vi "Add to Query.vi"(8 "error in (no error)":errorcluster, 9 "value":string, 10 "key":string, 11 "URI in":refnum<class "URI.lvclass">) -> (0 "error out":errorcluster, 3 "URI out":refnum<class "URI.lvclass">)   [LabVIEW 2013, in "openURI.lvlib" / "URI.lvclass"]
uses:
  URI.lvclass
  URI.lvclass/URI.ctl
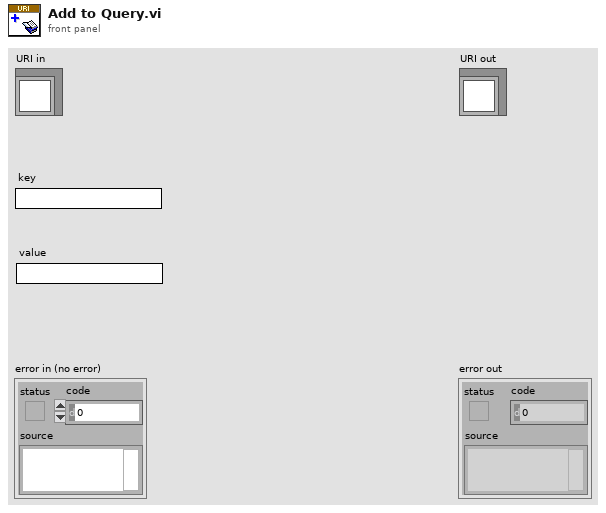
[diagram p1: front panel]
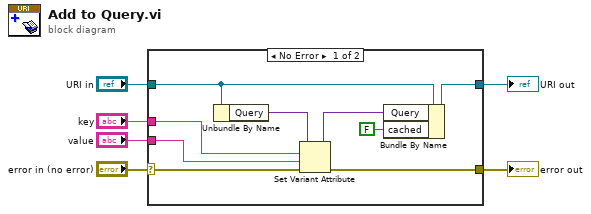
[diagram p0: block diagram]
diagram:
  n1 = case shown="No Error" "error in (no error)" {
    selector: "error in (no error)" -> [w9 w17]
    tunnel: [w8 w17] -> w5
    tunnel: [w12 w16] -> w3
    tunnel: "URI in" -> [w7 w16]
    tunnel: "key" -> [w15 _]
    tunnel: "value" -> [w14 _]
    frame No Error {
      n2 = Unbundle By Name(w7) -> ("Query"=w11:variant)
      n3 = Set Variant Attribute(Variant=w11, name=w15, value=w14, error in=w9) -> (Variant out=w13:variant, error out=w8:errorcluster)  [unwired: 1 out]
      n4 = Bundle By Name(cluster=w7, "Query"=w13, "cached"=FALSE) -> (w12:refnum<class "URI.lvclass">)
    }
    frame Error {
    }
  }
  "error out" <- w5
  "URI out" <- w3
